vi "LAbo2.3.vi"() -> ()   [LabVIEW 2020]
panel:
  out "x2:":string
  out "x1:":string
  out "x2:":dbl
  out "x1:":dbl
  out "ile pierwiastkow trojmianu kwadratowego:":string
  in  "Wartość c:":dbl
  in  "Wartość b:":dbl
  in  "Wartość a:":dbl
  out "wzór ogólny:":string
  out "Opis działania programu:":string caption="Opis działania programu"
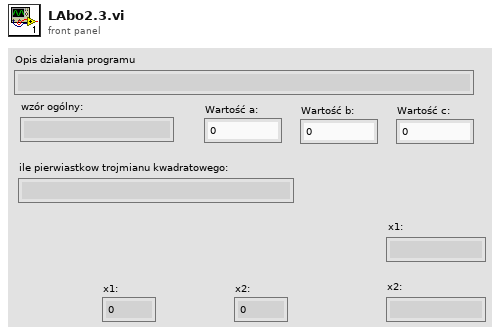
[diagram p1: front panel]
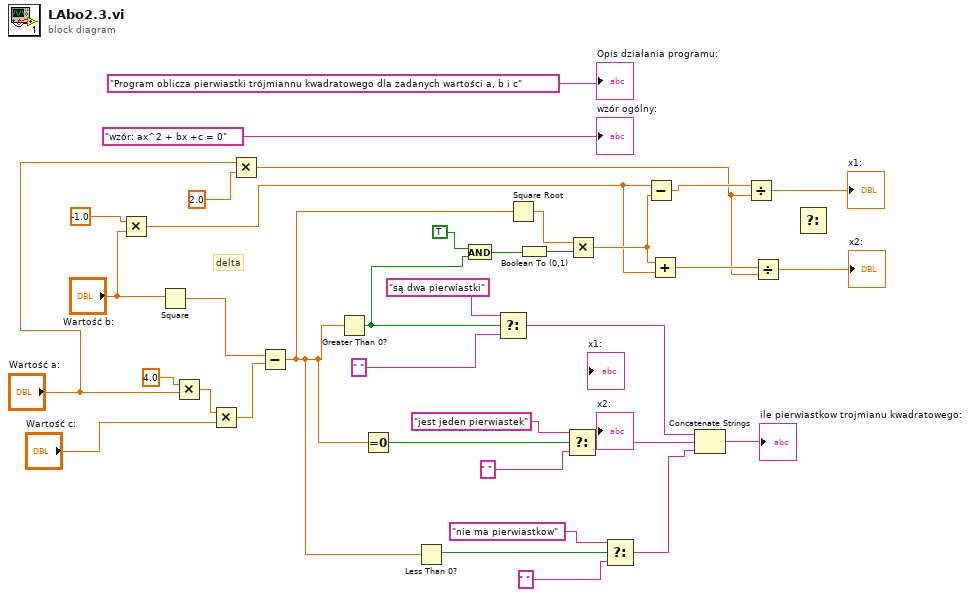
[diagram p0: block diagram]
diagram:
  # "delta"
  n1 = Multiply(x=-1.0, y="Wartość b:") -> (x*y=w8:dbl)
  n2 = Square(x="Wartość b:") -> (x^2=w18:dbl)
  n3 = Multiply(x=4.0, y="Wartość a:") -> (x*y=w32:dbl)
  n4 = Multiply(x=w32, y="Wartość c:") -> (x*y=w31:dbl)
  n5 = Multiply(x="Wartość a:", y=2.0) -> (x*y=w3:dbl)
  n6 = Subtract(x=w18, y=w31) -> (x-y=w13:dbl)
  n7 = Greater Than 0?(x=w13) -> (x > 0?=w17:bool)
  n8 = Equal To 0?(x=w13) -> (x = 0?=w28:bool)
  n9 = Less Than 0?(x=w13) -> (x < 0?=w23:bool)
  n10 = And(x=TRUE, y=w17) -> (x .and. y?=w15:bool)
  n11 = Select(t="są dwa pierwiastki", s=w17, f=" ") -> (s? t:f=w19:string)
  n12 = Square Root(x=w13) -> (sqrt(x)=w12:dbl)
  n13 = Boolean To (0,1)(Boolean=w15) -> (0, 1=w14:i16)
  n14 = Select(t="jest jeden pierwiastek", s=w28, f=" ") -> (s? t:f=w22:string)
  n15 = Multiply(x=w12, y=w14) -> (x*y=w9:dbl)
  n16 = Select(t="nie ma pierwiastkow", s=w23, f=" ") -> (s? t:f=w21:string)
  n17 = Subtract(x=w8, y=w9) -> (x-y=w5:dbl)
  n18 = Add(x=w9, y=w8) -> (x+y=w4:dbl)
  n19 = Concatenate Strings(w19, w22, w21) -> (→"ile pierwiastkow trojmianu kwadratowego:":string)
  n20 = Divide(x=w5, y=w3) -> (x/y=→"x1:":dbl)
  n21 = Divide(x=w4, y=w3) -> (x/y=→"x2:":dbl)
  n22 = Select() -> ()  [unwired: 3 in, 1 out]
  "Opis działania programu:" <- "Program oblicza pierwiastki trójmiannu kwadratowego dla zadanych wartości a, b i c"
  "wzór ogólny:" <- "wzór: ax^2 + bx +c = 0"
